vi "Update IP Address.vi"(8 "error in":errorcluster, 10 "Detected System":string, 11 "Package Name":string="//%s/CFX315") -> (0 "error out":errorcluster, 2 "Shared Variable Address":string, 3 "IP Address":string)   [LabVIEW 2019, in "GUI.lvlib"]
uses:
  GUI.lvlib
  <vilib>/regexp/Match Regular Expression.xnode
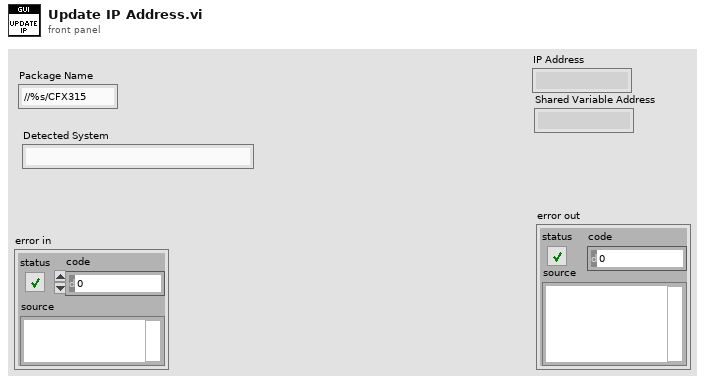
[diagram p1: front panel]
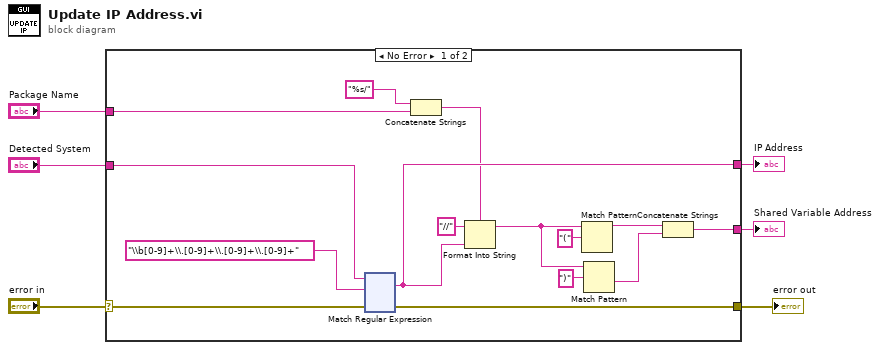
[diagram p0: block diagram]
diagram:
  n1 = case shown="No Error" "error in" {
    selector: "error in" -> [w15 w136]
    tunnel: [w14 w136] -> w5
    tunnel: "Detected System" -> [w13 _]
    tunnel: [w12 _] -> w3
    tunnel: [w11 _] -> w2
    tunnel: "Package Name" -> [w8 _]
    frame No Error {
      n2 = xnode "Match Regular Expression"("input string"=w13, "regular expression"="\\b[0-9]+\\.[0-9]+\\.[0-9]+\\.[0-9]+", "error in"=w15) -> ("whole match"=w12:string, "error out"=w14:errorcluster)  [unwired: 3 in, 3 out]
      n3 = Concatenate Strings("%s/" ("string"), w8) -> (w7:string)
      n4 = Format Into String(format string=w7, initial string="//", w12) -> (resulting string=w18:string)  [unwired: 1 in, 1 out]
      n5 = Match Pattern(string=w18, regular expression="(") -> (before substring=w20:string)  [unwired: 1 in, 3 out]
      n6 = Match Pattern(string=w18, regular expression=")") -> (after substring=w21:string)  [unwired: 1 in, 3 out]
      n7 = Concatenate Strings(w20, w21) -> (w11:string)
    }
    frame Error {
    }
  }
  "error out" <- w5
  "IP Address" <- w3
  "Shared Variable Address" <- w2
